vi "Report Unsupported Operating System.vi"(8 "error in (no error)":errorcluster) -> (0 "error out":errorcluster)   [LabVIEW 2018, in "Chassis TimeSync Engine.lvlib"]
uses:
  Chassis TimeSync Engine.lvlib
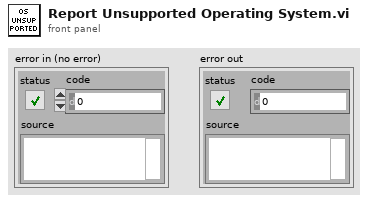
[diagram p1: front panel]
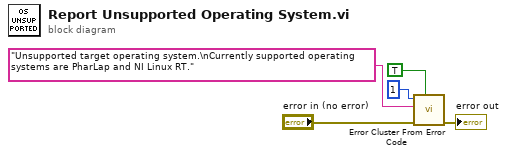
[diagram p0: block diagram]
diagram:
  n1 = call <vilib>:"Error Cluster From Error Code.vi"("show call chain? (False)"=TRUE, "error in (no error)"="error in (no error)", "error message (\"\")"="Unsupported target operating system.\nCurrently supported operating systems are PharLap and NI Linux RT." ("error message (\"\")"), "error code (0)"=1) -> ("error out"=→"error out":errorcluster)  [unwired: 5 in]
